vi "SCMP FITS - Make Single FITS Header.vi"(6 "FITS info":T4={"File name"="lsob_demo_0530_LM_20190529_124525_live_C1_00020_001_lev0.0.fits", "Date"="2019-05-29T12:45:25"}, 7 "Andor":T1={"Handle"=0, "Pixel Encoding"="", "AOI Width"=0, "AOI Height"=0, "AOI Stride"=0, "Row Readout Time"=0.0, "Frame Readout Time"=0.0, "Interframe Time"=0.0, "Semaphore"=refnum, "SerialNumber"="", "Camera Model"="", "Controller ID"="", "Firmware Version"="", "Shutter"="Global", "BDiv"=1, "Time at Synch"=timestamp(3029526000.379448 s since 1904-01-01), "Idx"=0, "PreAmp"="", "Binning"=enum."1x1", "PixelReadoutRate"="", "Exposure (s)"=0.05, "Image Bytes"=0, "Image Pixels"=0, "SpuriousNoiseFilter"=FALSE, "Overlap"=FALSE, "CycleMode"=""} {"Exposure (s)" format="%^.3g"; "Time at Synch" format="%<%H:%M:%S>T"; "Interframe Time" format="%#_3g"; "Frame Readout Time" format="%_3g"; "Row Readout Time" format="%_3g"}, 8 "error in":errorcluster, 9 "NAXIS":string="2", 10 "FITS Header":T5={"Wavelength (nm)"=530.15, "Exposure (s)"=0.05, "Tuning Delay (ms)"=1000.0, "Beam Type (-1/1)"=1.0, "Tuning Voltages"=[1.111, 2.222, 3.333, 4.444], "Observer"="observer", "Light Shapping Diffuser"=enum."In Beam", "Comment"="", "Data Type"=enum."HOLE", "Mod Cycles"=0, "SCD Calibration Optics"=enum."1 - Polarizer @0, I+Q", "SCD Emission Line Filter"=enum."1-557.6nm", "Cookbook"="", "COMP-S Calibration Wheel"=enum."Dark", "COMP-S Andover Filter Wheel"=enum."530.3nm/HWB 0.34nm (Fe XIV)", "FOV Rotation (deg)"=66.0, "Objective Lens Position (mm)"=0.0, "Occulter size"=0.0, "Time End"=timestamp(3382374145.421875 s since 1904-01-01), "Acc Exposure (s)"=0.0, "Time Stamp Array"=[], "Camera Serial Number"=[], "Camera Temp"=[], "Camera PI (mm)"=[], "Time Start"=timestamp(3382374145.421875 s since 1904-01-01), "Peripherals"={"ILX controler"=FALSE, "Zone temperatures"=FALSE, "Andor"=FALSE, "Andor 2"=FALSE, "PI Stages"=FALSE, "AISAS mechanisms"=FALSE, "AISAS Mech.lvclass"=refnum, "Zone temp ref"=variant, "FWs"=FALSE}, "FITS paths"=[], "Cameras"=enum."Andor", "load preset cbk"=FALSE, "periodic check count"=0, "COMP-S Calibration Wheel 2"=enum."Dark", "Calib"=enum."Dark", "Abso Aperture"=66.0, "Nominal Aperture"=66.0} {"Nominal Aperture" format="%.1f"; "Abso Aperture" format="%.1f"; "Camera PI (mm)" format="%_3g"; "Acc Exposure (s)" format="%^.3g"; "Occulter size" format="%.2f"; "Objective Lens Position (mm)" min=70.0 max=152.0 format="%.2f"; "FOV Rotation (deg)" format="%.1f"; "Exposure (s)" format="%^.3g"; "Wavelength (nm)" format="%_6g"}, 11 "Image #":i32) -> (0 "error out":errorcluster, 1 "23040 Byte Header":string="SIMPLE  =                              T / CONFORMS TO FITS STANDARD            BITPIX  =                             32 / BITS PER PIXEL                       NAXIS   =                              2 / DATA DIMENSIONS IN FITS FILE         NAXIS1  =                              0 / XDIM (PIXELS)                        NAXIS2  =                              0 / YDIM (PIXELS)                        NAXIS3  =                              4 / 4 POLARIZATION STATES                NAXIS4  =                              1 / 1 CAMERA                             ORIGIN  =                        'AISAS' / SCIENTIFIC GROUP                     OBSERVER=                     'SCHWARTZ' / NAME OF OBSERVER                     TELESCOP=                   '20CM ZEISS' / NAME OF TELESCOPE                    LOCATION=            'LOMNICKY PEAK OBS' / LOCATION OF TELESCOPE                INSTRUME=                          'SCD' / NAME OF INSTRUMENT                   BZERO   =                             0. /  ADU OFFSET                          FOCUS   =                             26 / CAMERA-STAGE POSITION (MM)           ROTPOS  =                           66.0 / ROTATIONAL POSITION (DEG)            DIFFUSER=                      'IN BEAM' / 0=IN BEAM, 1=OUT OF BEAM             FW-WVLNG=                        '557.6' / PRE-FILTER CENTER WAVELENGTH (NM)    FW-CALIB=                         'DARK' / CAL-WHEEL POSITION                   CAM-SN1 =                    'SCC-02209' / CAMERA SERIAL NUMBER                 CAM-TEMP=                       0.000000 / FOCAL PLANE TEMP (C)                 TUNEDLAY=                           1000 / LCVR RELAXATION DELAY (mS)           DATE_OBS=                     '3/7/2011' / DATE OF OBSERVATION START (UTC)      TIME_OBS=                   '212225.421' / TIME OF OBSERVATION (UTC)            EXPOSURE=                       0.050000 / EXPOSURE TIME (S)                    MODC    =                              0 / NUMBER OF IMAGES AT EACH STATE       NLC-1   =                          1.111 / TUNING VOLTAGE-1                     NLC-2   =                          2.222 / TUNING VOLTAGE-2                     NLC-3   =                          3.333 / TUNING VOLTAGE-3                     NLC-4   =                          4.444 / TUNING VOLTAGE-4                     NLC-5   =                          0.000 / TUNING VOLTAGE-5                     BEAM    =                              1 / BEAM (0=ON BAND OR 1=CONTINUUM)      WAVELENG=                         530.15 / WAVELENGTH OF OBS (NM)               COMMHEAD=                             '' / OBSERVER COMMENT                     COOKBOOK=                                / COOKBOOK  LOADED                     COMMENT                                                                         COMMENT                                                                         COMMENT                                                                         COMMENT                                                                         COMMENT                                                                         COMMENT                                                                         COMMENT                                                                         COMMENT                                                                         COMMENT                                                                         COMMENT                                                                         COMMENT                                                                         COMMENT                                                                         COMMENT                                                                         COMMENT                                                                         COMMENT                                                                         COMMENT                                                                         COMMENT                                                                         COMMENT                                                                         COMMENT                                                                         COMMENT                                                                         COMMENT                                                                         COMMENT                                                                         COMMENT                                                                         COMMENT                                                                         COMMENT                                                                         COMMENT                                                                         COMMENT                                                                         COMMENT                                                                         COMMENT                                                                         COMMENT                                                                         COMMENT                                                                         COMMENT                                                                         COMMENT                                                                         COMMENT                                                                         COMMENT                                                                         COMMENT                                                                         COMMENT                                                                         COMMENT                                                                         COMMENT                                                                         COMMENT                                                                         COMMENT                                                                         COMMENT                                                                         COMMENT                                                                         COMMENT                                                                         COMMENT                                                                         COMMENT                                                                         COMMENT                                                                         COMMENT                                                                         COMMENT                                                                         COMMENT                                                                         COMMENT                                                                         COMMENT                                                                         COMMENT                                                                         COMMENT                                                                         COMMENT                                                                         COMMENT                                                                         COMMENT                                                                         COMMENT                                                                         COMMENT                                                                         COMMENT                                                                         COMMENT                                                                         COMMENT                                                                         COMMENT                                                                         COMMENT                                                                         COMMENT                                                                         COMMENT                                                                         COMMENT                                                                         COMMENT                                                                         COMMENT                                                                         COMMENT                                                                         COMMENT                                                                         COMMENT                                                                         COMMENT                                                                         COMMENT                                                                         COMMENT                                                                         COMMENT                                                                         COMMENT                                                                         COMMENT                                                                         COMMENT                                                                         COMMENT                                                                         COMMENT                                                                         COMMENT                                                                         COMMENT                                                                         COMMENT                                                                         COMMENT                                                                         COMMENT                                                                         COMMENT                                                                         COMMENT                                                                         COMMENT                                                                         COMMENT                                                                         COMMENT                                                                         COMMENT                                                                         COMMENT                                                                         COMMENT                                                                         COMMENT                                                                         COMMENT                                                                         COMMENT                                                                         COMMENT                                                                         COMMENT                                                                         COMMENT                                                                         COMMENT                                                                         COMMENT                                                                         COMMENT                                                                         COMMENT                                                                         COMMENT                                                                         COMMENT                                                                         COMMENT                                                                         COMMENT                                                                         COMMENT                                                                         COMMENT                                                                         COMMENT                                                                         COMMENT                                                                         COMMENT                                                                         COMMENT                                                                         COMMENT                                                                         COMMENT                                                                         COMMENT                                                                         COMMENT                                                                         COMMENT                                                                         COMMENT                                                                         COMMENT                                                                         COMMENT                                                                         COMMENT                                                                         COMMENT                                                                         COMMENT                                                                         COMMENT                                                                         COMMENT                                                                         COMMENT                                                                         COMMENT                                                                         COMMENT                                                                         COMMENT                                                                         COMMENT                                                                         COMMENT                                                                         COMMENT                                                                         COMMENT                                                                         COMMENT                                                                         COMMENT                                                                         COMMENT                                                                         COMMENT                                                                         COMMENT                                                                         COMMENT                                                                         COMMENT                                                                         COMMENT                                                                         COMMENT                                                                         COMMENT                                                                         COMMENT                                                                         COMMENT                                                                         COMMENT                                                                         COMMENT                                                                         COMMENT                                                                         COMMENT                                                                         COMMENT                                                                         COMMENT                                                                         COMMENT                                                                         COMMENT                                                                         COMMENT                                                                         COMMENT                                                                         COMMENT                                                                         COMMENT                                                                         COMMENT                                                                         COMMENT                                                                         COMMENT                                                                         COMMENT                                                                         COMMENT                                                                         COMMENT                                                                         COMMENT                                                                         COMMENT                                                                         COMMENT                                                                         COMMENT                                                                         COMMENT                                                                         COMMENT                                                                         COMMENT                                                                         COMMENT                                                                         COMMENT                                                                         COMMENT                                                                         COMMENT                                                                         COMMENT                                                                         COMMENT                                                                         COMMENT                                                                         COMMENT                                                                         COMMENT                                                                         COMMENT                                                                         COMMENT                                                                         COMMENT                                                                         COMMENT                                                                         COMMENT                                                                         COMMENT                                                                         COMMENT                                                                         COMMENT                                                                         COMMENT                                                                         COMMENT                                                                         COMMENT                                                                         COMMENT                                                                         COMMENT                                                                         COMMENT                                                                         COMMENT                                                                         COMMENT                                                                         COMMENT                                                                         COMMENT                                                                         COMMENT                                                                         COMMENT                                                                         COMMENT                                                                         COMMENT                                                                         COMMENT                                                                         COMMENT                                                                         COMMENT                                                                         COMMENT                                                                         COMMENT                                                                         COMMENT                                                                         COMMENT                                                                         COMMENT                                                                         COMMENT                                                                         COMMENT                                                                         COMMENT                                                                         COMMENT                                                                         COMMENT                                                                         COMMENT                                                                         COMMENT                                                                         COMMENT                                                                         COMMENT                                                                         COMMENT                                                                         COMMENT                                                                         COMMENT                                                                         COMMENT                                                                         COMMENT                                                                         COMMENT                                                                         COMMENT                                                                         COMMENT                                                                         COMMENT                                                                         COMMENT                                                                         COMMENT                                                                         COMMENT                                                                         COMMENT                                                                         COMMENT                                                                         COMMENT                                                                         COMMENT                                                                         COMMENT                                                                         COMMENT                                                                         COMMENT                                                                         COMMENT                                                                         COMMENT                                                                         COMMENT                                                                         COMMENT                                                                         COMMENT                                                                         COMMENT                                                                         COMMENT                                                                         COMMENT                                                                         COMMENT                                                                         COMMENT                                                                         COMMENT                                                                         COMMENT                                                                         COMMENT                                                                         COMMENT                                                                         END                                                                             ", 3 "final header byte length":i32=23040)   [LabVIEW 2014]
uses:
  Controls/SCD - FITS Cluster.ctl
  AISAS/Mech/AISAS Mech.lvclass
  AISAS/Controls/Diffuser.ctl
  Controls/FITS Data type.ctl
  Controls/SCD - Calibration Optics Filter Wheel.ctl
  Controls/SCD - EDT - Emission Line Filter Wheel.ctl
  Controls/CoMP-S Controls/Polarization Optics Filter Wheel.ctl
  Controls/CoMP-S Controls/Emission Line Filter Wheel.ctl
  AISAS/Controls/focus.ctl
  Controls/peripherals.ctl
  Controls/Cameras select.ctl
  Controls/Fits info.ctl
  Camera/Andor Neo Info.ctl
  Controls/beaning.ctl
  Controls/Globals.vi
panel:
  out "Required COMMENT Rows":i32
  in  "NAXIS2":string="2160"
  in  "NAXIS1":string="2560"
  out "Header Rows":i32=34
  out "FITS Header":string[](array[string])=["SIMPLE  =                              T / CONFORMS TO FITS STANDARD            ", "BITPIX  =                             32 / BITS PER PIXEL                       ", "NAXIS   =                              2 / DATA DIMENSIONS IN FITS FILE         ", "NAXIS1  =                              0 / XDIM (PIXELS)                        ", "NAXIS2  =                              0 / YDIM (PIXELS)                        ", "NAXIS3  =                              4 / 4 POLARIZATION STATES                ", "NAXIS4  =                              1 / 1 CAMERA                             ", "ORIGIN  =                        'AISAS' / SCIENTIFIC GROUP                     ", "OBSERVER=                     'SCHWARTZ' / NAME OF OBSERVER                     ", "TELESCOP=                   '20CM ZEISS' / NAME OF TELESCOPE                    ", "LOCATION=            'LOMNICKY PEAK OBS' / LOCATION OF TELESCOPE                ", "INSTRUME=                          'SCD' / NAME OF INSTRUMENT                   ", "BZERO   =                             0. /  ADU OFFSET                          ", "FOCUS   =                             26 / CAMERA-STAGE POSITION (MM)           ", "ROTPOS  =                           66.0 / ROTATIONAL POSITION (DEG)            ", "DIFFUSER=                      'IN BEAM' / 0=IN BEAM, 1=OUT OF BEAM             ", "FW-WVLNG=                        '557.6' / PRE-FILTER CENTER WAVELENGTH (NM)    ", "FW-CALIB=                         'DARK' / CAL-WHEEL POSITION                   ", "CAM-SN1 =                    'SCC-02209' / CAMERA SERIAL NUMBER                 ", "CAM-TEMP=                       0.000000 / FOCAL PLANE TEMP (C)                 ", "TUNEDLAY=                           1000 / LCVR RELAXATION DELAY (mS)           ", "DATE_OBS=                     '3/7/2011' / DATE OF OBSERVATION START (UTC)      ", "TIME_OBS=                   '212225.421' / TIME OF OBSERVATION (UTC)            ", "EXPOSURE=                       0.050000 / EXPOSURE TIME (S)                    ", "MODC    =                              0 / NUMBER OF IMAGES AT EACH STATE       ", "NLC-1   =                          1.111 / TUNING VOLTAGE-1                     ", "NLC-2   =                          2.222 / TUNING VOLTAGE-2                     ", "NLC-3   =                          3.333 / TUNING VOLTAGE-3                     ", "NLC-4   =                          4.444 / TUNING VOLTAGE-4                     ", "NLC-5   =                          0.000 / TUNING VOLTAGE-5                     ", "BEAM    =                              1 / BEAM (0=ON BAND OR 1=CONTINUUM)      ", "WAVELENG=                         530.15 / WAVELENGTH OF OBS (NM)               ", "COMMHEAD=                             '' / OBSERVER COMMENT                     ", "COOKBOOK=                                / COOKBOOK  LOADED                     ", "COMMENT                                                                         ", "COMMENT                                                                         ", "COMMENT                                                                         ", "COMMENT                                                                         ", "COMMENT                                                                         ", "COMMENT                                                                         ", "COMMENT                                                                         ", "COMMENT                                                                         ", "COMMENT                                                                         ", "COMMENT                                                                         ", "COMMENT                                                                         ", "COMMENT                                                                         ", "COMMENT                                                                         ", "COMMENT                                                                         ", "COMMENT                                                                         ", "COMMENT                                                                         ", "COMMENT                                                                         ", "COMMENT                                                                         ", "COMMENT                                                                         ", "COMMENT                                                                         ", "COMMENT                                                                         ", "COMMENT                                                                         ", "COMMENT                                                                         ", "COMMENT                                                                         ", "COMMENT                                                                         ", "COMMENT                                                                         ", "COMMENT                                                                         ", "COMMENT                                                                         ", "COMMENT                                                                         ", "COMMENT                                                                         ", "COMMENT                                                                         ", "COMMENT                                                                         ", "COMMENT                                                                         ", "COMMENT                                                                         ", "COMMENT                                                                         ", "COMMENT                                                                         ", "COMMENT                                                                         ", "COMMENT                                                                         ", "COMMENT                                                                         ", "COMMENT                                                                         ", "COMMENT                                                                         ", "COMMENT                                                                         ", "COMMENT                                                                         ", "COMMENT                                                                         ", "COMMENT                                                                         ", "COMMENT                                                                         ", "COMMENT                                                                         ", "COMMENT                                                                         ", "COMMENT                                                                         ", "COMMENT                                                                         ", "COMMENT                                                                         ", "COMMENT                                                                         ", "COMMENT                                                                         ", "COMMENT                                                                         ", "COMMENT                                                                         ", "COMMENT                                                                         ", "COMMENT                                                                         ", "COMMENT                                                                         ", "COMMENT                                                                         ", "COMMENT                                                                         ", "COMMENT                                                                         ", "COMMENT                                                                         ", "COMMENT                                                                         ", "COMMENT                                                                         ", "COMMENT                                                                         ", "COMMENT                                                                         ", "COMMENT                                                                         ", "COMMENT                                                                         ", "COMMENT                                                                         ", "COMMENT                                                                         ", "COMMENT                                                                         ", "COMMENT                                                                         ", "COMMENT                                                                         ", "COMMENT                                                                         ", "COMMENT                                                                         ", "COMMENT                                                                         ", "COMMENT                                                                         ", "COMMENT                                                                         ", "COMMENT                                                                         ", "COMMENT                                                                         ", "COMMENT                                                                         ", "COMMENT                                                                         ", "COMMENT                                                                         ", "COMMENT                                                                         ", "COMMENT                                                                         ", "COMMENT                                                                         ", "COMMENT                                                                         ", "COMMENT                                                                         ", "COMMENT                                                                         ", "COMMENT                                                                         ", "COMMENT                                                                         ", "COMMENT                                                                         ", "COMMENT                                                                         ", "COMMENT                                                                         ", "COMMENT                                                                         ", "COMMENT                                                                         ", "COMMENT                                                                         ", "COMMENT                                                                         ", "COMMENT                                                                         ", "COMMENT                                                                         ", "COMMENT                                                                         ", "COMMENT                                                                         ", "COMMENT                                                                         ", "COMMENT                                                                         ", "COMMENT                                                                         ", "COMMENT                                                                         ", "COMMENT                                                                         ", "COMMENT                                                                         ", "COMMENT                                                                         ", "COMMENT                                                                         ", "COMMENT                                                                         ", "COMMENT                                                                         ", "COMMENT                                                                         ", "COMMENT                                                                         ", "COMMENT                                                                         ", "COMMENT                                                                         ", "COMMENT                                                                         ", "COMMENT                                                                         ", "COMMENT                                                                         ", "COMMENT                                                                         ", "COMMENT                                                                         ", "COMMENT                                                                         ", "COMMENT                                                                         ", "COMMENT                                                                         ", "COMMENT                                                                         ", "COMMENT                                                                         ", "COMMENT                                                                         ", "COMMENT                                                                         ", "COMMENT                                                                         ", "COMMENT                                                                         ", "COMMENT                                                                         ", "COMMENT                                                                         ", "COMMENT                                                                         ", "COMMENT                                                                         ", "COMMENT                                                                         ", "COMMENT                                                                         ", "COMMENT                                                                         ", "COMMENT                                                                         ", "COMMENT                                                                         ", "COMMENT                                                                         ", "COMMENT                                                                         ", "COMMENT                                                                         ", "COMMENT                                                                         ", "COMMENT                                                                         ", "COMMENT                                                                         ", "COMMENT                                                                         ", "COMMENT                                                                         ", "COMMENT                                                                         ", "COMMENT                                                                         ", "COMMENT                                                                         ", "COMMENT                                                                         ", "COMMENT                                                                         ", "COMMENT                                                                         ", "COMMENT                                                                         ", "COMMENT                                                                         ", "COMMENT                                                                         ", "COMMENT                                                                         ", "COMMENT                                                                         ", "COMMENT                                                                         ", "COMMENT                                                                         ", "COMMENT                                                                         ", "COMMENT                                                                         ", "COMMENT                                                                         ", "COMMENT                                                                         ", "COMMENT                                                                         ", "COMMENT                                                                         ", "COMMENT                                                                         ", "COMMENT                                                                         ", "COMMENT                                                                         ", "COMMENT                                                                         ", "COMMENT                                                                         ", "COMMENT                                                                         ", "COMMENT                                                                         ", "COMMENT                                                                         ", "COMMENT                                                                         ", "COMMENT                                                                         ", "COMMENT                                                                         ", "COMMENT                                                                         ", "COMMENT                                                                         ", "COMMENT                                                                         ", "COMMENT                                                                         ", "COMMENT                                                                         ", "COMMENT                                                                         ", "COMMENT                                                                         ", "COMMENT                                                                         ", "COMMENT                                                                         ", "COMMENT                                                                         ", "COMMENT                                                                         ", "COMMENT                                                                         ", "COMMENT                                                                         ", "COMMENT                                                                         ", "COMMENT                                                                         ", "COMMENT                                                                         ", "COMMENT                                                                         ", "COMMENT                                                                         ", "COMMENT                                                                         ", "COMMENT                                                                         ", "COMMENT                                                                         ", "COMMENT                                                                         ", "COMMENT                                                                         ", "COMMENT                                                                         ", "COMMENT                                                                         ", "COMMENT                                                                         ", "COMMENT                                                                         ", "COMMENT                                                                         ", "COMMENT                                                                         ", "COMMENT                                                                         ", "COMMENT                                                                         ", "COMMENT                                                                         ", "COMMENT                                                                         ", "COMMENT                                                                         ", "COMMENT                                                                         ", "COMMENT                                                                         ", "COMMENT                                                                         ", "COMMENT                                                                         ", "COMMENT                                                                         ", "COMMENT                                                                         ", "COMMENT                                                                         ", "COMMENT                                                                         ", "COMMENT                                                                         ", "COMMENT                                                                         ", "COMMENT                                                                         ", "COMMENT                                                                         ", "COMMENT                                                                         ", "COMMENT                                                                         ", "COMMENT                                                                         ", "COMMENT                                                                         ", "COMMENT                                                                         ", "COMMENT                                                                         ", "COMMENT                                                                         ", "COMMENT                                                                         ", "COMMENT                                                                         ", "COMMENT                                                                         ", "COMMENT                                                                         ", "COMMENT                                                                         ", "COMMENT                                                                         ", "COMMENT                                                                         ", "COMMENT                                                                         ", "COMMENT                                                                         ", "COMMENT                                                                         ", "COMMENT                                                                         ", "COMMENT                                                                         ", "COMMENT                                                                         ", "COMMENT                                                                         ", "COMMENT                                                                         ", "COMMENT                                                                         ", "COMMENT                                                                         ", "COMMENT                                                                         ", "COMMENT                                                                         ", "COMMENT                                                                         ", "COMMENT                                                                         ", "COMMENT                                                                         ", "COMMENT                                                                         ", "END                                                                             "]
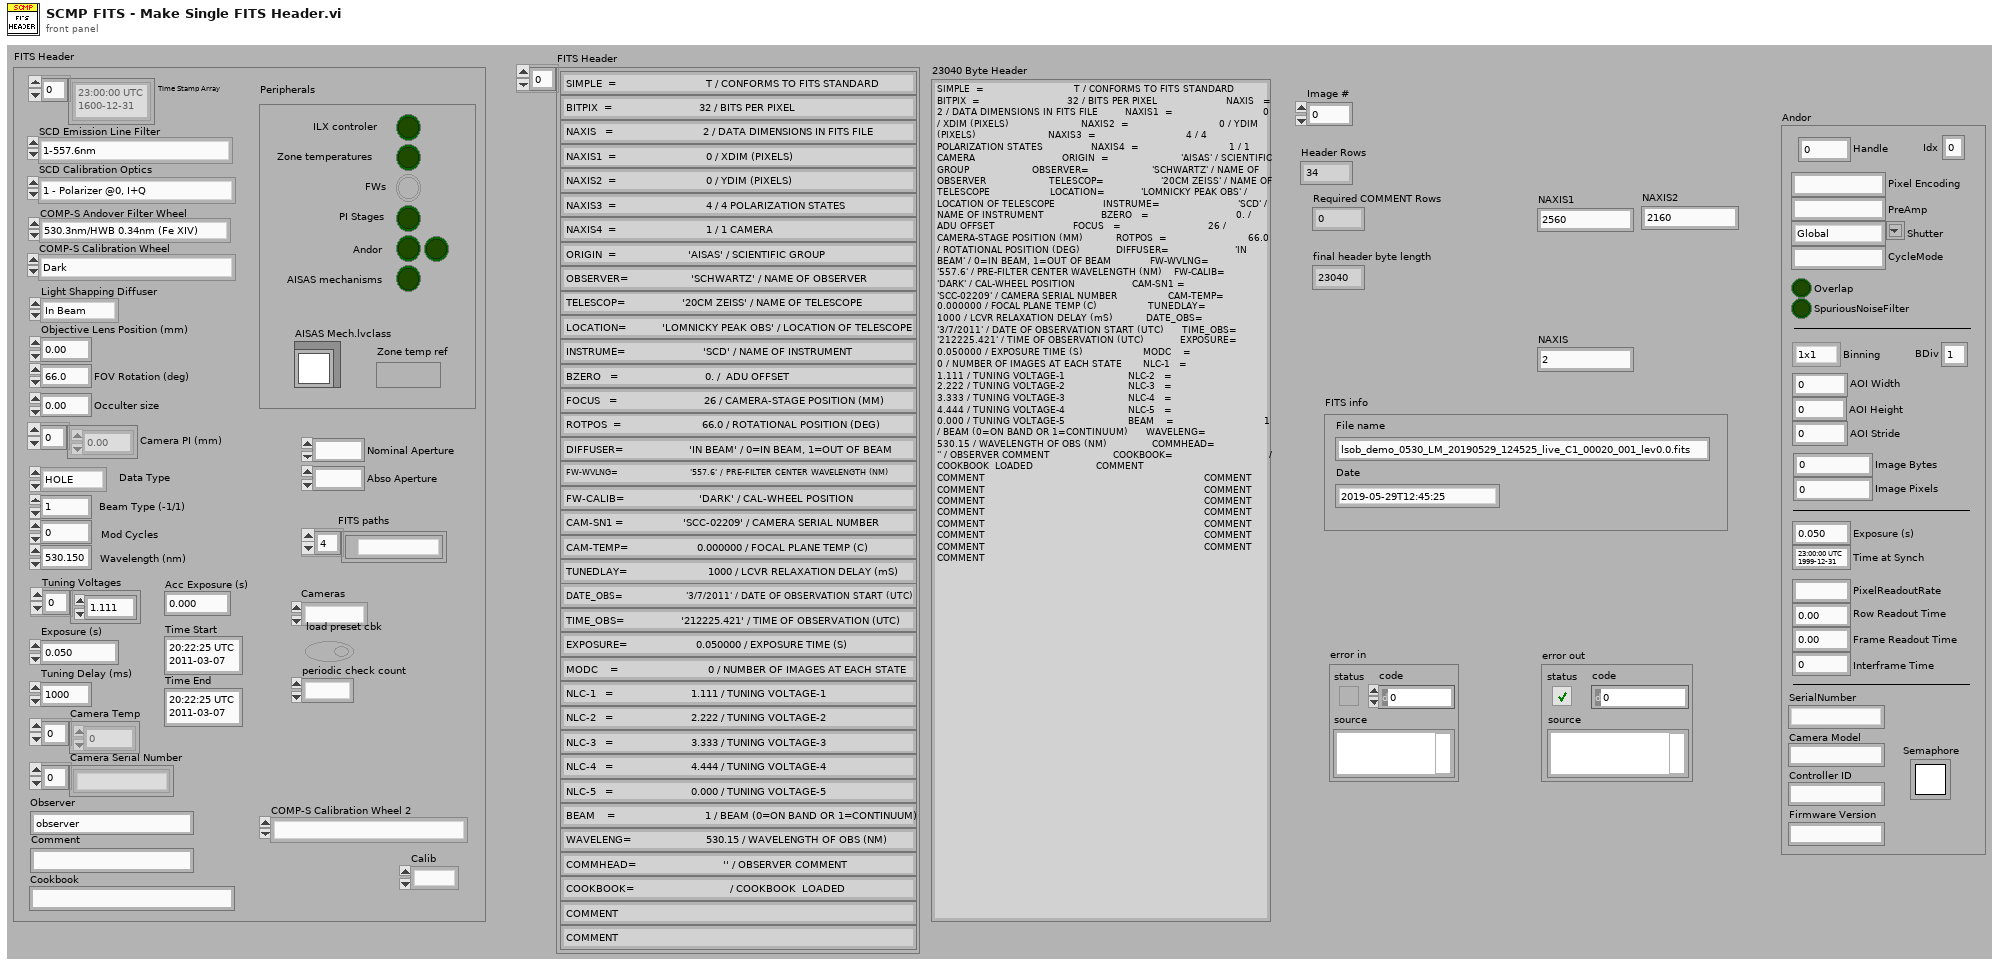
[diagram p1: front panel]
types:
  T1 = typedef "Andor Neo Info.ctl" = cluster{"Handle":i32, "Pixel Encoding":string, "AOI Width":i32, "AOI Height":i32, "AOI Stride":i32, "Row Readout Time":dbl, "Frame Readout Time":dbl, "Interframe Time":dbl, "Semaphore":T2, "SerialNumber":string, "Camera Model":string, "Controller ID":string, "Firmware Version":string, "Shutter":string, "BDiv":u8, "Time at Synch":timestamp, "Idx":i32, "PreAmp":string, "Binning":T3, "PixelReadoutRate":string, "Exposure (s)":dbl, "Image Bytes":i64, "Image Pixels":i64, "SpuriousNoiseFilter":bool, "Overlap":bool, "CycleMode":string}
  T2 = typedef "Semaphore RefNum" = refnum<k1>
  T3 = typedef "beaning.ctl" = enum16{"1x1", "2x2", "3x3", "4x4", "8x8"}
  T4 = typedef "Fits info.ctl" = cluster{"File name":string, "Date":string}
  T5 = typedef "SCD - FITS Cluster.ctl" = cluster{"Wavelength (nm)":dbl, "Exposure (s)":dbl, "Tuning Delay (ms)":dbl, "Beam Type (-1/1)":dbl, "Tuning Voltages":dbl[], "Observer":string, "Light Shapping Diffuser":T6, "Comment":string, "Data Type":T7, "Mod Cycles":u16, "SCD Calibration Optics":T8, "SCD Emission Line Filter":T9, "Cookbook":string, "COMP-S Calibration Wheel":T10, "COMP-S Andover Filter Wheel":T11, "FOV Rotation (deg)":dbl, "Objective Lens Position (mm)":T12, "Occulter size":dbl, "Time End":timestamp, "Acc Exposure (s)":dbl, "Time Stamp Array":timestamp[], "Camera Serial Number":string[], "Camera Temp":dbl[], "Camera PI (mm)":dbl[], "Time Start":timestamp, "Peripherals":T13, "FITS paths":path[], "Cameras":T14, "load preset cbk":bool, "periodic check count":i32, "COMP-S Calibration Wheel 2":T10, "Calib":enum16{"Dark", "Flat"}, "Abso Aperture":dbl, "Nominal Aperture":dbl}
  T6 = typedef "Diffuser.ctl" = enum16{"Out of Beam", "In Beam"}
  T7 = typedef "FITS Data type.ctl" = enum16{"LIVE", "DARK", "FLAT", "CALI", "OBSE", "ABSO", "AURE", "TARG", "OBJE", "HOLE", "OREX", "THRO", "CHIP"}
  T8 = typedef "SCD - Calibration Optics Filter Wheel.ctl" = enum16{"1 - Polarizer @0, I+Q", "2 - Polarizer @90, I-Q", "3 - Polarizer @45, I+U", "4 - Polarizer @135, I-U", "5 - Polarizer @0, Retarder @45, I+V", "6 - Polarizer @0, Retarder @135, I-V", "7 - Dark", "8 - Clear", "9 - N/A"}
  T9 = typedef "SCD - EDT - Emission Line Filter Wheel.ctl" = enum16{"1-557.6nm", "2-587.6nm", "3-589.6nm", "4-630.2nm", "5-656.4nm", "6-849.8nm", "7-854.2nm", "8-866.2nm", "9-1083.0nm"}
  T10 = typedef "Polarization Optics Filter Wheel.ctl" = enum16{"Dark", "Clear", "Exchange Lens", "Polarizer @0, I+Q", "Polarizer @90, I-Q", "Polarizer @45, I+U", "Polarizer @135, I-U", "Polarizer @0, Retarder @45, I+V", "Polarizer @0, Retarder @135, I-V"}
  T11 = typedef "Emission Line Filter Wheel.ctl" = enum16{"530.3nm/HWB 0.34nm (Fe XIV)", "587.6nm/HBW 0.44nm (He I D3)", "637.5nm/HBW 0.53nm (Fe X)", "656.3nm/HBW 0.57nm (H-Alpha)", "789.2nm/HBW 0.85nm (Fe XI)", "854.2nm/HBW 1.01nm (Ca I)", "1074.7nm/HBW 2.34nm (Fe XIII)", "1079.8nm/HBW 1.64nm (Fe XIII)", "1083.0nm/HBW 1.66nm (He I)"}
  T12 = typedef "focus.ctl" = dbl
  T13 = typedef "peripherals.ctl" = cluster{"ILX controler":bool, "Zone temperatures":bool, "Andor":bool, "Andor 2":bool, "PI Stages":bool, "AISAS mechanisms":bool, "AISAS Mech.lvclass":refnum<class "AISAS Mech.lvclass">, "Zone temp ref":variant, "FWs":bool}
  T14 = typedef "Cameras select.ctl" = enum16{"Andor", "GDR"}
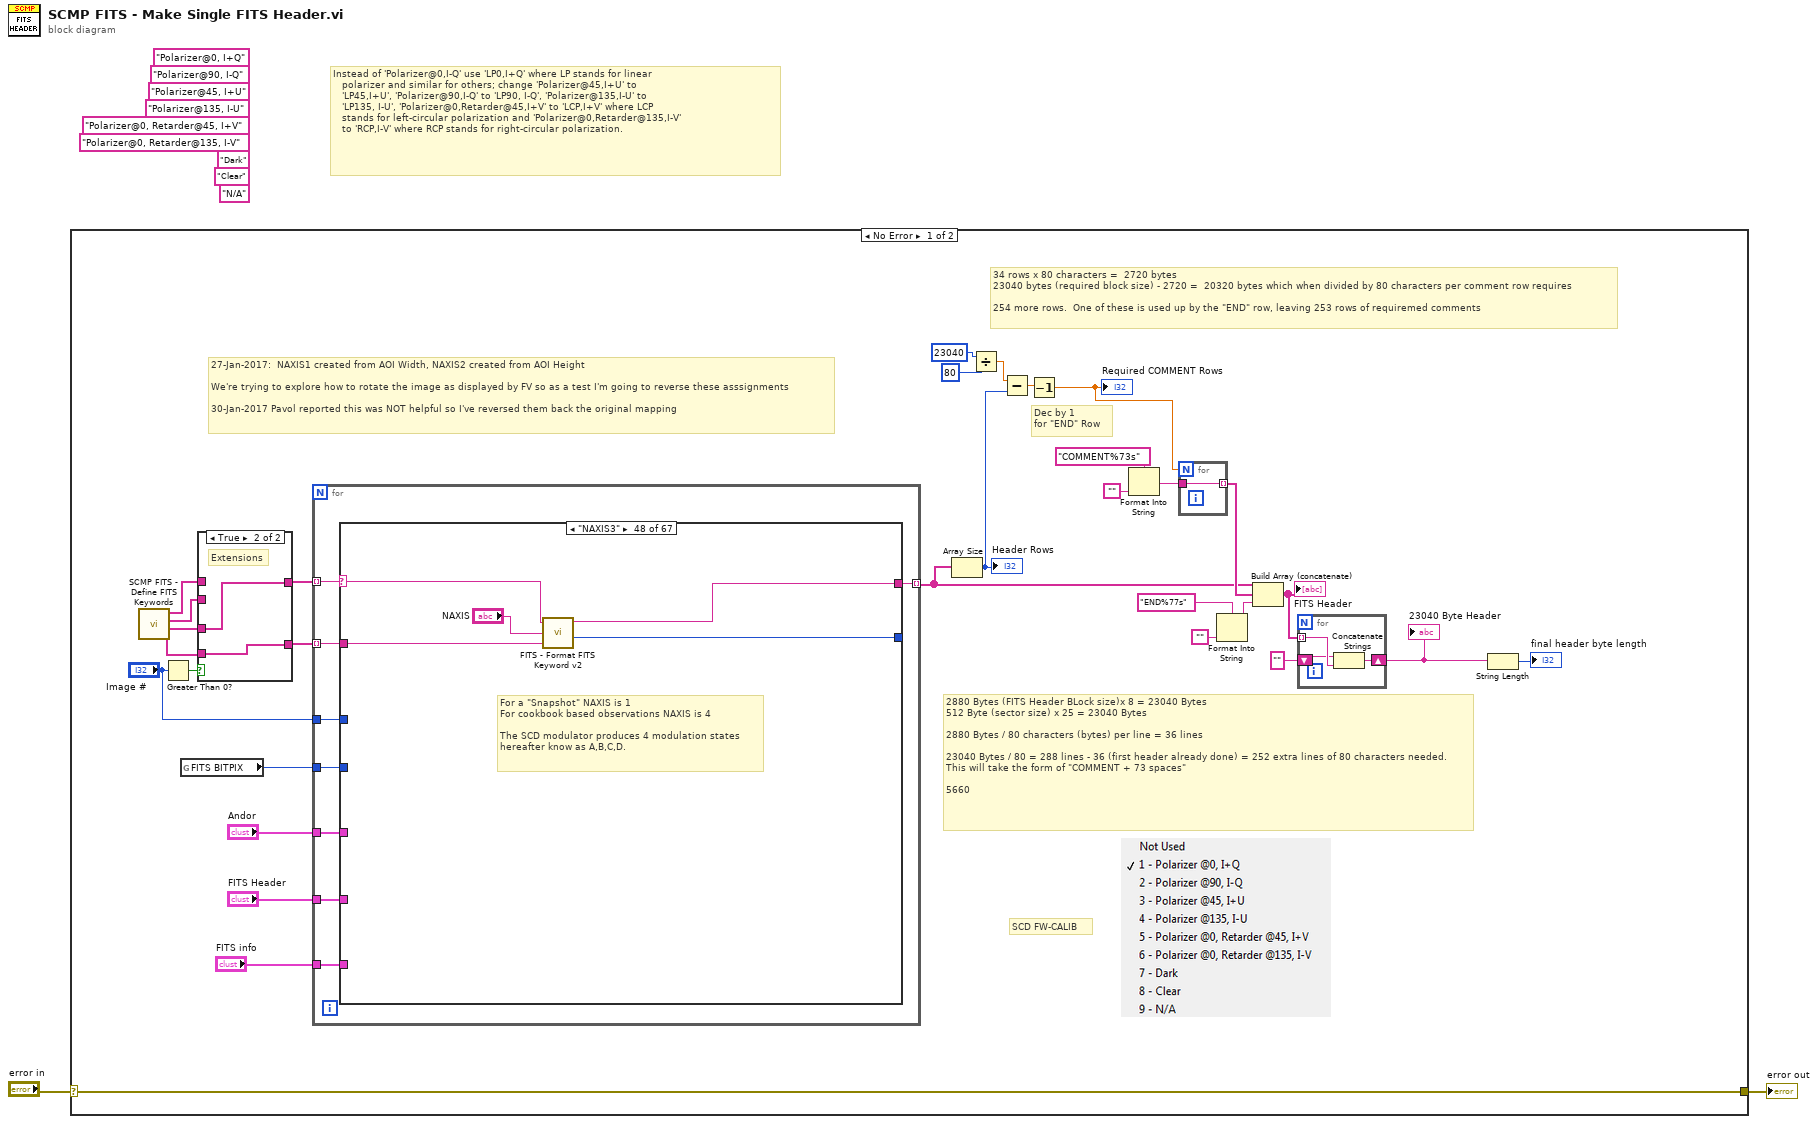
[diagram p0: block diagram]
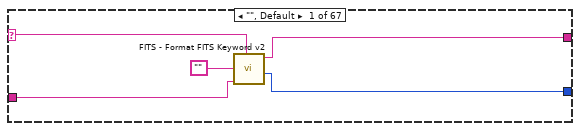
[diagram p3: hidden frame]
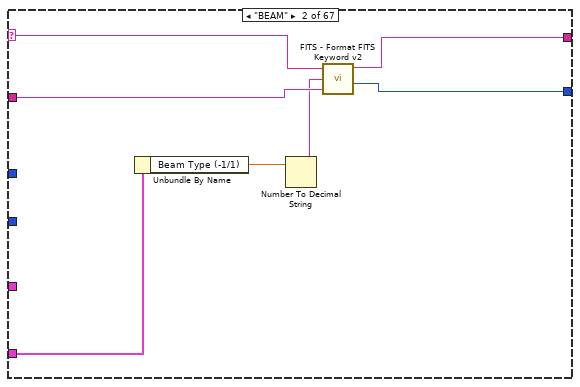
[diagram p4: hidden frame]
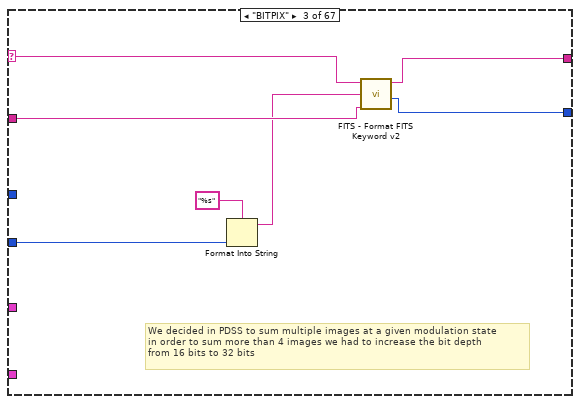
[diagram p5: hidden frame]
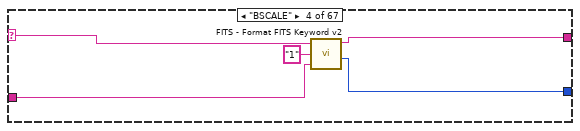
[diagram p6: hidden frame]
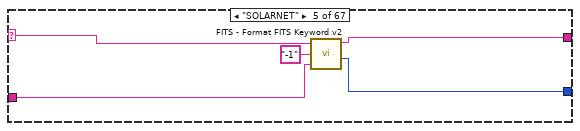
[diagram p7: hidden frame]
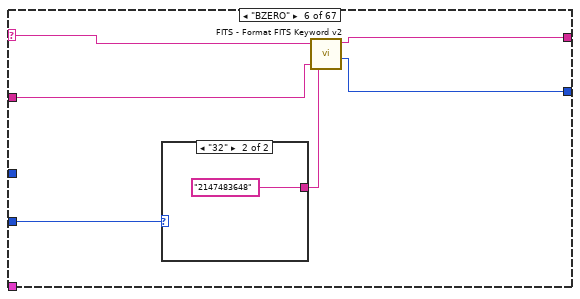
[diagram p8: hidden frame]
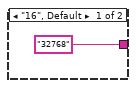
[diagram p9: hidden frame]
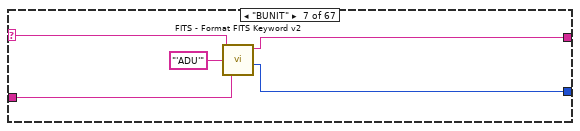
[diagram p10: hidden frame]
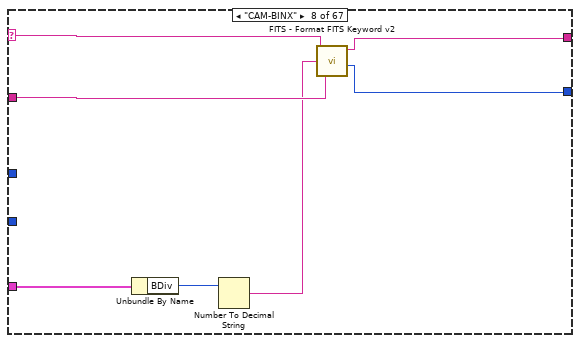
[diagram p11: hidden frame]
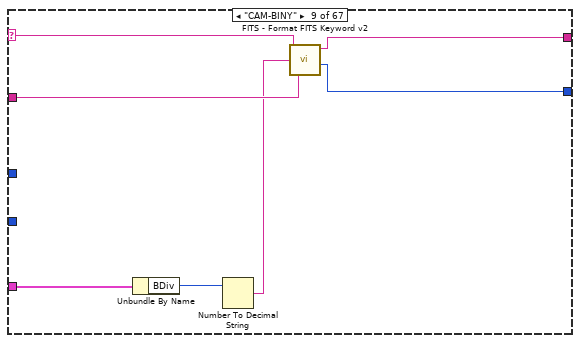
[diagram p12: hidden frame]
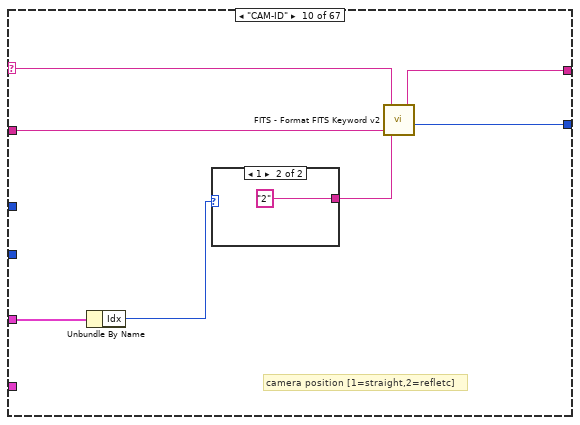
[diagram p13: hidden frame]
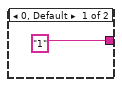
[diagram p14: hidden frame]
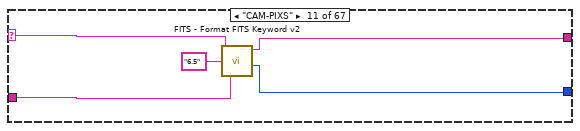
[diagram p15: hidden frame]
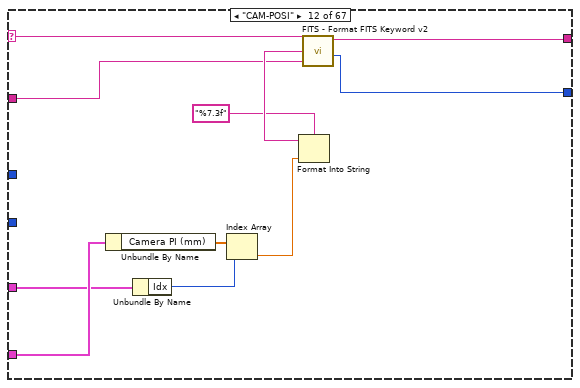
[diagram p16: hidden frame]
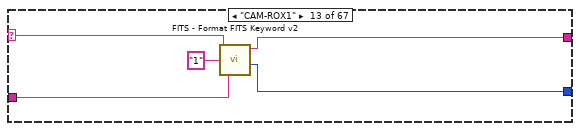
[diagram p17: hidden frame]
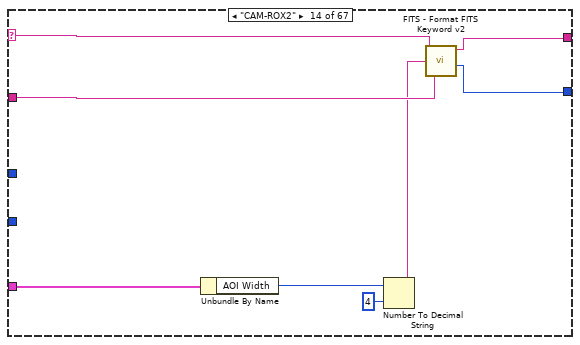
[diagram p18: hidden frame]
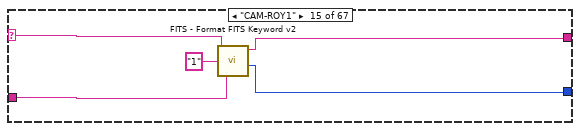
[diagram p19: hidden frame]
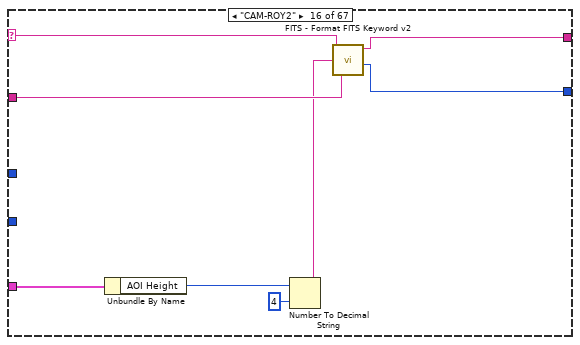
[diagram p20: hidden frame]
diagram:
  (unwired) "N/A" ("element")
  (unwired) "Clear" ("element")
  (unwired) "Dark" ("element")
  (unwired) "Polarizer@0, Retarder@135, I-V" ("element")
  (unwired) "Polarizer@0, Retarder@45, I+V" ("element")
  (unwired) "Polarizer@135, I-U" ("element")
  (unwired) "Polarizer@45, I+U"
  (unwired) "Polarizer@90, I-Q"
  (unwired) "Polarizer@0, I+Q"
  # "Instead of 'Polarizer@0,I-Q' use 'LP0,I+Q' where LP stands for linear\n   polarizer and similar for others; change 'Polarizer@45,I+U' to\n   'LP45,I+U', 'Polarizer@90,I-Q' to 'LP90, I-Q', 'Polarizer@135,I-U' to\n   'LP135, I-U', 'Polarizer@0,Retarder@45,I+V' to 'LCP,I+V' where LCP\n   stands for left-circular polarization and 'Polarizer@0,Retarder@135,I-V'\n   to 'RCP,I-V' where RCP stands for right-circular polarization."
  n1 = case shown="No Error" "error in" {
    selector: "error in" -> [w14 w605]
    tunnel: [w14 w605] -> w1
    frame No Error {
      # "SCD FW-CALIB"
      # "27-Jan-2017:  NAXIS1 created from AOI Width, NAXIS2 created from AOI Height\n\nWe're trying to explore how to rotate the image as displayed by FV so as a test I'm going to reverse these asssignments\n\n30-Jan-2017 Pavol reported this was NOT helpful so I've reversed them back the original mapping"
      # "34 rows x 80 characters =  2720 bytes\n23040 bytes (required block size) - 2720 =  20320 bytes which when divided by 80 characters per comment row requires\n\n254 more rows.  One of these is used up by the \"END\" row, leaving 253 rows of requiremed comments"
      # "Dec by 1\nfor \"END\" Row"
      # "2880 Bytes (FITS Header BLock size)x 8 = 23040 Bytes\n512 Byte (sector size) x 25 = 23040 Bytes\n\n2880 Bytes / 80 characters (bytes) per line = 36 lines\n\n23040 Bytes / 80 = 288 lines - 36 (first header already done) = 252 extra lines of 80 characters needed.\nThis will take the form of \"COMMENT + 73 spaces\" \n\n5660"
      n2 = call "SCMP FITS - Define FITS Keywords.vi"() -> ("Extension Comments"=w26:string[], "Extension  Keywords"=w27:string[], "Primary Comments"=w28:string[], "Primary Keywords"=w25:string[])  [unwired: 5 in, 3 out]
      n3 = Greater Than 0?(x="Image #") -> (x > 0?=w31:bool)
      n4 = global read "Globals.vi" "FITS BITPIX"() -> (w5:enum16{"16", "32"})
      n5 = case shown="True" w31 {
        tunnel: [w39 w41] -> w30
        tunnel: [w38 w40] -> w29
        tunnel: w25 -> [w39 _]
        tunnel: w28 -> [w38 _]
        tunnel: w27 -> [_ w41]
        tunnel: w26 -> [_ w40]
        frame False {
          # "Primary"
        }
        frame True {
          # "Extensions"
        }
      }
      n6 = for {
        tunnel: w30 -> [w44] mode=indexing
        tunnel: w29 -> [w48] mode=indexing
        tunnel: "FITS Header" -> [w49]
        tunnel: [w47] -> w13 mode=indexing
        tunnel: "Andor" -> [w46]
        tunnel: "Image #" -> [w45]
        tunnel: w5 -> [w43]
        tunnel: "FITS info" -> [w42]
        n7 = case shown="\"NAXIS3\"" w44 {
          selector: w44 -> [w54 w61 w68 w73 w78 w84 w90 w98 w105 w112 w118 w128 w134 w143 w147 w156 w167 w178 w184 w191 w199 w220 w227 w242 w254 w260 w268 w278 w289 w300 w310 w315 w323 w328 w335 w339 w347 w356 w388 w393 w398 w405 w409 w416 w424 w442 w449 w463 w468 w478 w488 w498 w508 w518 w526 w534 w541 w547 w552 w556 w565 w570 w574 w580 w591 w596 w603]
          tunnel: w49 -> [_ w58 _ _ _ _ _ _ _ _ _ w122 _ _ _ _ w164 w172 w180 w192 w200 _ w224 w244 w252 w258 w270 w276 _ w297 w307 _ _ _ _ _ w344 w353 w384 _ _ _ _ w413 _ _ _ _ _ w475 w485 w495 w505 w515 w522 w532 w538 _ _ w560 _ _ _ w577 w588 _ w599]
          tunnel: w48 -> [w52 w60 w67 w72 w77 w83 w89 w97 w104 w111 w117 w127 w133 w142 w146 w155 w166 w177 w183 w190 w198 w219 w226 w243 w253 w259 w269 w277 w288 w299 w309 w314 w322 w327 w334 w338 w346 w355 w387 w391 w397 w403 w408 w415 w423 w441 w450 w462 w467 w477 w487 w497 w507 w517 w525 w533 w540 w546 w550 w557 w564 w569 w573 w579 w590 w595 w602]
          tunnel: [w51 w59 w66 w71 w76 w82 w87 w96 w103 w110 w116 w126 w132 w141 w145 w154 w165 w176 w182 w189 w197 w218 w225 w240 w251 w257 w267 w279 w287 w298 w308 w313 w321 w326 w332 w337 w345 w354 w386 w390 w396 w404 w407 w414 w422 w440 w448 w461 w466 w476 w486 w496 w506 w516 w524 w530 w539 w545 w549 w555 w563 w568 w572 w578 w589 w594 w601] -> w47
          tunnel: [w50 w55 w65 w70 w75 w81 w88 w95 w102 w109 w115 w125 w131 w140 w144 w153 w163 w174 w181 w188 w196 w217 w222 w241 w250 w256 w266 w280 w286 w296 w304 w311 w320 w325 w333 w336 w342 w352 w385 w389 w395 w402 w406 w411 w421 w439 w447 w460 w464 w474 w484 w494 w504 w514 w523 w531 w536 w544 w548 w554 w561 w567 w571 w576 w584 w592 w600] -> _
          tunnel: w46 -> [_ _ _ _ _ _ _ w94 w101 w107 _ w121 _ w136 _ w150 w158 w169 _ _ _ _ _ _ _ _ _ _ _ _ _ _ _ _ _ _ _ _ _ _ _ _ _ _ _ w436 w451 _ _ _ _ _ _ _ _ _ _ _ _ _ _ _ _ _ _ _ _]
          tunnel: w45 -> [_ _ _ _ _ _ _ _ _ _ _ _ _ _ _ _ _ _ _ _ _ _ _ _ _ _ _ _ _ _ _ _ _ _ _ _ _ _ _ _ _ _ _ _ w419 _ _ _ _ _ _ _ _ _ _ _ _ _ _ _ _ _ _ _ _ _ _]
          tunnel: w43 -> [_ _ w64 _ _ w79 _ _ _ _ _ _ _ _ _ _ _ _ _ _ _ _ _ _ _ _ _ _ _ _ _ _ _ _ _ _ _ _ _ _ _ _ _ _ _ _ _ _ _ _ _ _ _ _ _ _ _ _ _ _ _ _ _ _ _ _ _]
          tunnel: w42 -> [_ _ _ _ _ _ _ _ _ _ _ _ _ _ _ _ _ _ _ _ _ w215 w221 _ _ _ _ _ _ _ _ _ w319 _ _ _ _ _ _ _ _ _ _ _ _ _ _ _ _ _ _ _ _ _ _ _ _ _ _ _ _ _ _ _ _ _ _]
          frame "", Default {
            n8 = call "FITS - Format FITS Keyword v2 .vi"("Keyword"=w54, "Value"="", "Comment"=w52) -> ("Formatted fits entry"=w51:string, "Length of line"=w50:i16)  [unwired: 1 in, 1 out]
          }
          frame "BEAM" {
            n9 = Unbundle By Name(w58) -> ("Beam Type (-1/1)"=w56:dbl)
            n10 = Number To Decimal String(number=w56) -> (decimal integer string=w57:string)  [unwired: 1 out]
            n11 = call "FITS - Format FITS Keyword v2 .vi"("Keyword"=w61, "Value"=w57, "Comment"=w60) -> ("Formatted fits entry"=w59:string, "Length of line"=w55:i16)  [unwired: 1 in, 1 out]
          }
          frame "BITPIX" {
            # "We decided in PDSS to sum multiple images at a given modulation state\nin order to sum more than 4 images we had to increase the bit depth\nfrom 16 bits to 32 bits"
            n12 = Format Into String(format string="%s", w64) -> (resulting string=w62:string)  [unwired: 2 in, 1 out]
            n13 = call "FITS - Format FITS Keyword v2 .vi"("Keyword"=w68, "Value"=w62, "Comment"=w67) -> ("Formatted fits entry"=w66:string, "Length of line"=w65:i16)  [unwired: 1 in, 1 out]
          }
          frame "BSCALE" {
            n14 = call "FITS - Format FITS Keyword v2 .vi"("Keyword"=w73, "Value"="1", "Comment"=w72) -> ("Formatted fits entry"=w71:string, "Length of line"=w70:i16)  [unwired: 1 in, 1 out]
          }
          frame "SOLARNET" {
            n15 = call "FITS - Format FITS Keyword v2 .vi"("Keyword"=w78, "Value"="-1", "Comment"=w77) -> ("Formatted fits entry"=w76:string, "Length of line"=w75:i16)  [unwired: 1 in, 1 out]
          }
          frame "BZERO" {
            n16 = case shown="\"32\"" w79 {
              tunnel: ["32768" ("Value") "2147483648" ("Value")] -> w80
              frame "16", Default {
              }
              frame "32" {
              }
            }
            n17 = call "FITS - Format FITS Keyword v2 .vi"("Keyword"=w84, "Value"=w80, "Comment"=w83) -> ("Formatted fits entry"=w82:string, "Length of line"=w81:i16)  [unwired: 1 in, 1 out]
          }
          frame "BUNIT" {
            n18 = call "FITS - Format FITS Keyword v2 .vi"("Keyword"=w90, "Value"="'ADU'", "Comment"=w89) -> ("Formatted fits entry"=w87:string, "Length of line"=w88:i16)  [unwired: 1 in, 1 out]
          }
          frame "CAM-BINX" {
            n19 = Unbundle By Name(w94) -> ("BDiv"=w93:u8)
            n20 = Number To Decimal String(number=w93) -> (decimal integer string=w92:string)  [unwired: 1 in]
            n21 = call "FITS - Format FITS Keyword v2 .vi"("Keyword"=w98, "Value"=w92, "Comment"=w97) -> ("Formatted fits entry"=w96:string, "Length of line"=w95:i16)  [unwired: 1 in, 1 out]
          }
          frame "CAM-BINY" {
            n22 = Unbundle By Name(w101) -> ("BDiv"=w99:u8)
            n23 = Number To Decimal String(number=w99) -> (decimal integer string=w100:string)  [unwired: 1 in]
            n24 = call "FITS - Format FITS Keyword v2 .vi"("Keyword"=w105, "Value"=w100, "Comment"=w104) -> ("Formatted fits entry"=w103:string, "Length of line"=w102:i16)  [unwired: 1 in, 1 out]
          }
          frame "CAM-ID" {
            # "camera position [1=straight,2=refletc]"
            n25 = Unbundle By Name(w107) -> ("Idx"=w106:i32)
            n26 = case shown="1" w106 {
              tunnel: ["1" ("string") "2" ("string")] -> w108
              frame 0, Default {
              }
              frame 1 {
              }
            }
            n27 = call "FITS - Format FITS Keyword v2 .vi"("Keyword"=w112, "Value"=w108, "Comment"=w111) -> ("Formatted fits entry"=w110:string, "Length of line"=w109:i16)  [unwired: 1 in, 1 out]
          }
          frame "CAM-PIXS" {
            n28 = call "FITS - Format FITS Keyword v2 .vi"("Keyword"=w118, "Value"="6.5", "Comment"=w117) -> ("Formatted fits entry"=w116:string, "Length of line"=w115:i16)  [unwired: 1 in, 1 out]
          }
          frame "CAM-POSI" {
            n29 = Unbundle By Name(w122) -> ("Camera PI (mm)"=w124:dbl[])
            n30 = Unbundle By Name(w121) -> ("Idx"=w123:i32)
            n31 = Index Array(array=w124, index=w123) -> (element=w120:dbl)
            n32 = Format Into String(format string="%7.3f", w120) -> (resulting string=w130:string)  [unwired: 2 in, 1 out]
            n33 = call "FITS - Format FITS Keyword v2 .vi"("Keyword"=w128, "Value"=w130, "Comment"=w127) -> ("Formatted fits entry"=w126:string, "Length of line"=w125:i16)  [unwired: 1 in, 1 out]
          }
          frame "CAM-ROX1" {
            n34 = call "FITS - Format FITS Keyword v2 .vi"("Keyword"=w134, "Value"="1", "Comment"=w133) -> ("Formatted fits entry"=w132:string, "Length of line"=w131:i16)  [unwired: 1 in, 1 out]
          }
          frame "CAM-ROX2" {
            n35 = Unbundle By Name(w136) -> ("AOI Width"=w138:i32)
            n36 = Number To Decimal String(number=w138, width (-)=i16 4) -> (decimal integer string=w137:string)
            n37 = call "FITS - Format FITS Keyword v2 .vi"("Keyword"=w143, "Value"=w137, "Comment"=w142) -> ("Formatted fits entry"=w141:string, "Length of line"=w140:i16)  [unwired: 1 in, 1 out]
          }
          frame "CAM-ROY1" {
            n38 = call "FITS - Format FITS Keyword v2 .vi"("Keyword"=w147, "Value"="1", "Comment"=w146) -> ("Formatted fits entry"=w145:string, "Length of line"=w144:i16)  [unwired: 1 in, 1 out]
          }
          frame "CAM-ROY2" {
            n39 = Unbundle By Name(w150) -> ("AOI Height"=w151:i32)
            n40 = Number To Decimal String(number=w151, width (-)=i16 4) -> (decimal integer string=w149:string)
            n41 = call "FITS - Format FITS Keyword v2 .vi"("Keyword"=w156, "Value"=w149, "Comment"=w155) -> ("Formatted fits entry"=w154:string, "Length of line"=w153:i16)  [unwired: 1 in, 1 out]
          }
          frame "CAM-SN" {
            w162 = "'" ("string")
            n42 = Unbundle By Name(w164) -> ("Camera Serial Number"=w160:string[])
            n43 = Unbundle By Name(w158) -> ("Idx"=w157:i32)
            n44 = Index Array(array=w160, index=w157) -> (element=w159:string)
            n45 = Concatenate Strings(w162, w159, w162) -> (w161:string)
            n46 = call "FITS - Format FITS Keyword v2 .vi"("Keyword"=w167, "Value"=w161, "Comment"=w166) -> ("Formatted fits entry"=w165:string, "Length of line"=w163:i16)  [unwired: 1 in, 1 out]
          }
          frame "CAM-TEMP" {
            n47 = Unbundle By Name(w169) -> ("Idx"=w168:i32)
            n48 = Unbundle By Name(w172) -> ("Camera Temp"=w171:dbl[])
            n49 = Index Array(array=w171, index=w168) -> (element=w170:dbl)
            n50 = Format Into String(format string="%6.2f", w170) -> (resulting string=w175:string)  [unwired: 2 in, 1 out]
            n51 = call "FITS - Format FITS Keyword v2 .vi"("Keyword"=w178, "Value"=w175, "Comment"=w177) -> ("Formatted fits entry"=w176:string, "Length of line"=w174:i16)  [unwired: 1 in, 1 out]
          }
          frame "COMMHEAD" {
            n52 = Unbundle By Name(w180) -> ("Comment"=w179:string)
            n53 = call "FITS - Format FITS Keyword v2 .vi"("Keyword"=w184, "Value"=w179, "Comment"=w183) -> ("Formatted fits entry"=w182:string, "Length of line"=w181:i16)  [unwired: 1 in, 1 out]
          }
          frame "COOKBOOK" {
            w187 = "'" ("string")
            n54 = Unbundle By Name(w192) -> ("Cookbook"=w186:string)
            n55 = Concatenate Strings(w187, w186, w187) -> (w185:string)
            n56 = call "FITS - Format FITS Keyword v2 .vi"("Keyword"=w191, "Value"=w185, "Comment"=w190) -> ("Formatted fits entry"=w189:string, "Length of line"=w188:i16)  [unwired: 1 in, 1 out]
          }
          frame "DATATYPE" {
            w195 = "'" ("string")
            n57 = disable-structure shown="Enabled" {
              disable-tunnel: w200 -> [w203 _]
              disable-tunnel: [w201 w214] -> w194
              frame Disabled {
                n58 = Unbundle By Name(w203) -> ("Data Type"=w202:T7)
                n59 = case shown="\"OBSE\"" w202 {
                  tunnel: ["DARK" "FLAT" "CALI" "OBSE" "ABSO" "AURE" "TARG" "OBJE" "HOLE" "LIVE"] -> w201
                  frame "LIVE", Default {
                  }
                  frame "DARK" {
                  }
                  frame "FLAT" {
                  }
                  frame "CALI" {
                  }
                  frame "OBSE" {
                  }
                  frame "ABSO" {
                  }
                  frame "AURE" {
                  }
                  frame "TARG" {
                  }
                  frame "OBJE" {
                  }
                  frame "HOLE" {
                  }
                }
              }
              frame Enabled {
                n60 = property on="Data Type" class="Enum (strict)"() -> ("RingText.Text"=w214:string)  [unwired: 2 in, 2 out]
              }
            }
            n61 = Concatenate Strings(w195, w194, w195) -> (w193:string)
            n62 = call "FITS - Format FITS Keyword v2 .vi"("Keyword"=w199, "Value"=w193, "Comment"=w198) -> ("Formatted fits entry"=w197:string, "Length of line"=w196:i16)  [unwired: 1 in, 1 out]
          }
          frame "DATE" {
            n63 = Unbundle By Name(w215) -> ("Date"=w216:string)
            n64 = call "FITS - Format FITS Keyword v2 .vi"("Keyword"=w220, "Value"=w216, "Comment"=w219) -> ("Formatted fits entry"=w218:string, "Length of line"=w217:i16)  [unwired: 1 in, 1 out]
          }
          frame "DATE-OBS" {
            # "FITS standard says that the DATE_OBS keyword is used for \nthe START of the observation"
            n65 = disable-structure shown="Enabled" {
              disable-tunnel: w224 -> [w229 w233]
              disable-tunnel: [w230 w236] -> w223
              disable-tunnel: w221 -> [_ _]
              frame Enabled {
                # "ten isty cas ako vo fits name"
                n66 = Unbundle By Name(w229) -> ("Time Start"=w228:timestamp)
                n67 = Format Date/Time String(time format string (%c)="%Y-%m-%dT%H:%M:%S", seconds (now)=w228) -> (date/time string=w230:string)  [unwired: 1 in]
              }
              frame Disabled {
                # "cas frame1 a zaokruhluje sa na sekundy"
                n68 = Unbundle By Name(w233) -> ("Time Stamp Array"=w234:timestamp[])
                n69 = Index Array(array=w234, index=0) -> (element=w232:timestamp)
                n70 = Format Date/Time String(time format string (%c)="%Y-%m-%dT%H:%M:%S", seconds (now)=w232) -> (date/time string=w236:string)  [unwired: 1 in]
              }
            }
            n71 = call "FITS - Format FITS Keyword v2 .vi"("Keyword"=w227, "Value"=w223, "Comment"=w226) -> ("Formatted fits entry"=w225:string, "Length of line"=w222:i16)  [unwired: 1 in, 1 out]
          }
          frame "DATE-END" {
            n72 = Unbundle By Name(w244) -> ("Time End"=w239:timestamp)
            n73 = Format Date/Time String(time format string (%c)="%Y-%m-%dT%H:%M:%S", seconds (now)=w239) -> (date/time string=w245:string)  [unwired: 1 in]
            n74 = call "FITS - Format FITS Keyword v2 .vi"("Keyword"=w242, "Value"=w245, "Comment"=w243) -> ("Formatted fits entry"=w240:string, "Length of line"=w241:i16)  [unwired: 1 in, 1 out]
          }
          frame "TIME-FR1" {
            n75 = Unbundle By Name(w252) -> ("Time Stamp Array"=w248:timestamp[])
            n76 = Index Array(array=w248, index=0) -> (element=w247:timestamp)
            n77 = Format Date/Time String(time format string (%c)="%H:%M:%S%3u", seconds (now)=w247) -> (date/time string=w255:string)  [unwired: 1 in]
            n78 = call "FITS - Format FITS Keyword v2 .vi"("Keyword"=w254, "Value"=w255, "Comment"=w253) -> ("Formatted fits entry"=w251:string, "Length of line"=w250:i16)  [unwired: 1 in, 1 out]
          }
          frame "TIME-FR2" {
            n79 = Unbundle By Name(w258) -> ("Time Stamp Array"=w263:timestamp[])
            n80 = Index Array(array=w263, index=1) -> (element=w262:timestamp)
            n81 = Format Date/Time String(time format string (%c)="%H:%M:%S%3u", seconds (now)=w262) -> (date/time string=w265:string)  [unwired: 1 in]
            n82 = call "FITS - Format FITS Keyword v2 .vi"("Keyword"=w260, "Value"=w265, "Comment"=w259) -> ("Formatted fits entry"=w257:string, "Length of line"=w256:i16)  [unwired: 1 in, 1 out]
          }
          frame "TIME-FR3" {
            n83 = Unbundle By Name(w270) -> ("Time Stamp Array"=w273:timestamp[])
            n84 = Index Array(array=w273, index=2) -> (element=w272:timestamp)
            n85 = Format Date/Time String(time format string (%c)="%H:%M:%S%3u", seconds (now)=w272) -> (date/time string=w275:string)  [unwired: 1 in]
            n86 = call "FITS - Format FITS Keyword v2 .vi"("Keyword"=w268, "Value"=w275, "Comment"=w269) -> ("Formatted fits entry"=w267:string, "Length of line"=w266:i16)  [unwired: 1 in, 1 out]
          }
          frame "TIME-FR4" {
            n87 = Unbundle By Name(w276) -> ("Time Stamp Array"=w283:timestamp[])
            n88 = Index Array(array=w283, index=3) -> (element=w282:timestamp)
            n89 = Format Date/Time String(time format string (%c)="%H:%M:%S%3u", seconds (now)=w282) -> (date/time string=w285:string)  [unwired: 1 in]
            n90 = call "FITS - Format FITS Keyword v2 .vi"("Keyword"=w278, "Value"=w285, "Comment"=w277) -> ("Formatted fits entry"=w279:string, "Length of line"=w280:i16)  [unwired: 1 in, 1 out]
          }
          frame "DETECTOR" {
            n91 = call "FITS - Format FITS Keyword v2 .vi"("Keyword"=w289, "Value"="'ANDOR NEO CAMERA'", "Comment"=w288) -> ("Formatted fits entry"=w287:string, "Length of line"=w286:i16)  [unwired: 1 in, 1 out]
          }
          frame "DIFFUSER" {
            n92 = Unbundle By Name(w297) -> ("Light Shapping Diffuser"=w294:T6)
            n93 = Build Array("'OUT OF BEAM'", "'IN BEAM'") -> (w295:string[])
            n94 = Index Array(array=w295, index=w294) -> (element=w293:string)
            n95 = call "FITS - Format FITS Keyword v2 .vi"("Keyword"=w300, "Value"=w293, "Comment"=w299) -> ("Formatted fits entry"=w298:string, "Length of line"=w296:i16)  [unwired: 1 in, 1 out]
          }
          frame "EXPTIME" {
            n96 = Unbundle By Name(w307) -> ("Exposure (s)"=w305:dbl)
            n97 = Multiply(x=1000.0, y=w305) -> (x*y=w302:dbl)
            n98 = Format Into String(format string="%_3f", w302) -> (resulting string=w306:string)  [unwired: 2 in, 1 out]
            n99 = call "FITS - Format FITS Keyword v2 .vi"("Keyword"=w310, "Value"=w306, "Comment"=w309) -> ("Formatted fits entry"=w308:string, "Length of line"=w304:i16)  [unwired: 1 in, 1 out]
          }
          frame "EXTEND" {
            n100 = call "FITS - Format FITS Keyword v2 .vi"("Keyword"=w315, "Value"="T", "Comment"=w314) -> ("Formatted fits entry"=w313:string, "Length of line"=w311:i16)  [unwired: 1 in, 1 out]
          }
          frame "FILENAME" {
            w318 = "'" ("string")
            n101 = Unbundle By Name(w319) -> ("File name"=w317:string)
            n102 = Concatenate Strings(w318, w317, w318) -> (w316:string)
            n103 = call "FITS - Format FITS Keyword v2 .vi"("Keyword"=w323, "Value"=w316, "Comment"=w322) -> ("Formatted fits entry"=w321:string, "Length of line"=w320:i16)  [unwired: 1 in, 1 out]
          }
          frame "FILTER" {
            n104 = disable-structure shown="SCMP==SCD" {
              disable-tunnel: ["'HAO Lyot 4-stage'" "'HAO Lyot 5-stage'"] -> w324
              frame condition #0 (active) {
              }
              frame condition #1 {
              }
            }
            n105 = call "FITS - Format FITS Keyword v2 .vi"("Keyword"=w328, "Value"=w324, "Comment"=w327) -> ("Formatted fits entry"=w326:string, "Length of line"=w325:i16)  [unwired: 1 in, 1 out]
          }
          frame "FLC-1" {
            n106 = call "FITS - Format FITS Keyword v2 .vi"("Keyword"=w335, "Value"="'+5.00,-5.00,+5.00,-5.00'", "Comment"=w334) -> ("Formatted fits entry"=w332:string, "Length of line"=w333:i16)  [unwired: 1 in, 1 out]
          }
          frame "FLC-2" {
            n107 = call "FITS - Format FITS Keyword v2 .vi"("Keyword"=w339, "Value"="'+5.00,-5.00,-5.00,+5.00'", "Comment"=w338) -> ("Formatted fits entry"=w337:string, "Length of line"=w336:i16)  [unwired: 1 in, 1 out]
          }
          frame "FOCUS" {
            n108 = Unbundle By Name(w344) -> ("Objective Lens Position (mm)"=w343:T12)
            n109 = Format Into String(format string="%5.2f", w343) -> (resulting string=w348:string)  [unwired: 2 in, 1 out]
            n110 = call "FITS - Format FITS Keyword v2 .vi"("Keyword"=w347, "Value"=w348, "Comment"=w346) -> ("Formatted fits entry"=w345:string, "Length of line"=w342:i16)  [unwired: 1 in, 1 out]
          }
          frame "FW-CALIB" {
            w351 = "'" ("string")
            n111 = disable-structure shown="SCMP==SCD" {
              disable-tunnel: w353 -> [w369 w382]
              disable-tunnel: [w367 w380] -> w350
              frame condition #0 {
                n112 = Unbundle By Name(w369) -> ("SCD Calibration Optics"=w368:T8)
                n113 = Build Array("LP0, I+Q", "LP90, I-Q", "LP45, I+U", "LP135, I-U" ("element"), "LCP, I+V" ("element"), "RCP, I-V" ("element"), "Dark" ("element"), "Clear" ("element"), "N/A" ("element")) -> (w357:string[])
                n114 = Index Array(array=w357, index=w368) -> (element=w367:string)
              }
              frame condition #1 (active) {
                n115 = Unbundle By Name(w382) -> ("COMP-S Calibration Wheel"=w381:T10)
                n116 = Build Array("Dark", "Clear", "Lens", "I+Q" ("element"), "I-Q" ("element"), "I+U" ("element"), "I-U" ("element"), "I+V" ("element"), "I-V" ("element")) -> (w372:string[])
                n117 = Index Array(array=w372, index=w381) -> (element=w380:string)
              }
            }
            n118 = Concatenate Strings(w351, w350, w351) -> (w349:string)
            n119 = call "FITS - Format FITS Keyword v2 .vi"("Keyword"=w356, "Value"=w349, "Comment"=w355) -> ("Formatted fits entry"=w354:string, "Length of line"=w352:i16)  [unwired: 1 in, 1 out]
          }
          frame "FW-WVLNG" {
            n120 = call "SCMP get wave from fw.vi"("FITS Header"=w384) -> ("element"=w383:string)  [unwired: 9 in, 1 out]
            n121 = call "FITS - Format FITS Keyword v2 .vi"("Keyword"=w388, "Value"=w383, "Comment"=w387) -> ("Formatted fits entry"=w386:string, "Length of line"=w385:i16)  [unwired: 1 in, 1 out]
          }
          frame "GCOUNT" {
            n122 = call "FITS - Format FITS Keyword v2 .vi"("Keyword"=w393, "Value"="1", "Comment"=w391) -> ("Formatted fits entry"=w390:string, "Length of line"=w389:i16)  [unwired: 1 in, 1 out]
          }
          frame "INSTRUME" {
            n123 = disable-structure shown="SCMP==SCD" {
              disable-tunnel: ["'COMP-S'" "'SCD'"] -> w394
              frame condition #0 (active) {
              }
              frame condition #1 {
              }
            }
            n124 = call "FITS - Format FITS Keyword v2 .vi"("Keyword"=w398, "Value"=w394, "Comment"=w397) -> ("Formatted fits entry"=w396:string, "Length of line"=w395:i16)  [unwired: 1 in, 1 out]
          }
          frame "LOCATION" {
            n125 = call "FITS - Format FITS Keyword v2 .vi"("Keyword"=w405, "Value"="'LOMNICKY PEAK OBSERVATORY'", "Comment"=w403) -> ("Formatted fits entry"=w404:string, "Length of line"=w402:i16)  [unwired: 1 in, 1 out]
          }
          frame "LEVEL" {
            n126 = call "FITS - Format FITS Keyword v2 .vi"("Keyword"=w409, "Value"="0", "Comment"=w408) -> ("Formatted fits entry"=w407:string, "Length of line"=w406:i16)  [unwired: 1 in, 1 out]
          }
          frame "MODC" {
            n127 = Unbundle By Name(w413) -> ("Mod Cycles"=w412:u16)
            n128 = Format Into String(format string="%d", w412) -> (resulting string=w417:string)  [unwired: 2 in, 1 out]
            n129 = call "FITS - Format FITS Keyword v2 .vi"("Keyword"=w416, "Value"=w417, "Comment"=w415) -> ("Formatted fits entry"=w414:string, "Length of line"=w411:i16)  [unwired: 1 in, 1 out]
          }
          frame "NAXIS" {
            n130 = Equal To 0?(x=w419) -> (x = 0?=w420:bool)
            n131 = case shown="False" w420 {
              tunnel: w424 -> [w427 w434]
              tunnel: w423 -> [w428 w433]
              tunnel: [w426 w432] -> w422
              tunnel: [w425 w431] -> w421
              frame False {
                # "All SCD Images have\n3 dimensions\nx-pixels\ny-pixels\npol state"
                n132 = call "FITS - Format FITS Keyword v2 .vi"("Keyword"=w427, "Value"="3", "Comment"=w428) -> ("Formatted fits entry"=w426:string, "Length of line"=w425:i16)  [unwired: 1 in, 1 out]
              }
              frame True {
                n133 = call "FITS - Format FITS Keyword v2 .vi"("Keyword"=w434, "Value"="0", "Comment"=w433) -> ("Formatted fits entry"=w432:string, "Length of line"=w431:i16)  [unwired: 1 in, 1 out]
              }
            }
          }
          frame "NAXIS1" {
            # "mh maj19 kamera na COMP-S je otocena o 90st\nmh jul19 -aj tak nakoniec netreba rotovat"
            n134 = disable-structure shown="SCMP==COMP, Default" {
              disable-tunnel: w436 -> [w444 w446]
              disable-tunnel: [w443 w445] -> w435
              frame condition #0 (active) {
                n135 = Unbundle By Name(w444) -> ("AOI Width"=w443:i32)
              }
              frame condition #1 {
                n136 = Unbundle By Name(w446) -> ("AOI Width"=w445:i32)
              }
            }
            n137 = Number To Decimal String(number=w435, width (-)=i16 4) -> (decimal integer string=w437:string)
            n138 = call "FITS - Format FITS Keyword v2 .vi"("Keyword"=w442, "Value"=w437, "Comment"=w441) -> ("Formatted fits entry"=w440:string, "Length of line"=w439:i16)  [unwired: 1 in, 1 out]
          }
          frame "NAXIS2" {
            # "mh maj19 kamera na COMP-S je otocena o 90st\nmh jul19 -aj tak nakoniec netreba rotovat"
            n139 = disable-structure shown="SCMP==COMP, Default" {
              disable-tunnel: w451 -> [w456 w458]
              disable-tunnel: [w455 w457] -> w452
              frame condition #0 (active) {
                n140 = Unbundle By Name(w456) -> ("AOI Height"=w455:i32)
              }
              frame condition #1 {
                n141 = Unbundle By Name(w458) -> ("AOI Height"=w457:i32)
              }
            }
            n142 = Number To Decimal String(number=w452, width (-)=i16 4) -> (decimal integer string=w453:string)
            n143 = call "FITS - Format FITS Keyword v2 .vi"("Keyword"=w449, "Value"=w453, "Comment"=w450) -> ("Formatted fits entry"=w448:string, "Length of line"=w447:i16)  [unwired: 1 in, 1 out]
          }
          frame "NAXIS3" {
            # "For a \"Snapshot\" NAXIS is 1\nFor cookbook based observations NAXIS is 4\n\nThe SCD modulator produces 4 modulation states\nhereafter know as A,B,C,D."
            n144 = call "FITS - Format FITS Keyword v2 .vi"("Keyword"=w463, "Value"="NAXIS", "Comment"=w462) -> ("Formatted fits entry"=w461:string, "Length of line"=w460:i16)  [unwired: 1 in, 1 out]
          }
          frame "NAXIS4" {
            # "SCD is a single camera instrument"
            n145 = call "FITS - Format FITS Keyword v2 .vi"("Keyword"=w468, "Value"="1", "Comment"=w467) -> ("Formatted fits entry"=w466:string, "Length of line"=w464:i16)  [unwired: 1 in, 1 out]
          }
          frame "NLC-1" {
            n146 = Unbundle By Name(w475) -> ("Tuning Voltages"=w471:dbl[])
            n147 = Index Array(array=w471, index=0) -> (element=w470:dbl)
            n148 = Format Into String(format string="%0.3f", w470) -> (resulting string=w469:string)  [unwired: 2 in, 1 out]
            n149 = call "FITS - Format FITS Keyword v2 .vi"("Keyword"=w478, "Value"=w469, "Comment"=w477) -> ("Formatted fits entry"=w476:string, "Length of line"=w474:i16)  [unwired: 1 in, 1 out]
          }
          frame "NLC-2" {
            n150 = Unbundle By Name(w485) -> ("Tuning Voltages"=w481:dbl[])
            n151 = Index Array(array=w481, index=1) -> (element=w480:dbl)
            n152 = Format Into String(format string="%0.3f", w480) -> (resulting string=w479:string)  [unwired: 2 in, 1 out]
            n153 = call "FITS - Format FITS Keyword v2 .vi"("Keyword"=w488, "Value"=w479, "Comment"=w487) -> ("Formatted fits entry"=w486:string, "Length of line"=w484:i16)  [unwired: 1 in, 1 out]
          }
          frame "NLC-3" {
            n154 = Unbundle By Name(w495) -> ("Tuning Voltages"=w491:dbl[])
            n155 = Index Array(array=w491, index=2) -> (element=w490:dbl)
            n156 = Format Into String(format string="%0.3f", w490) -> (resulting string=w489:string)  [unwired: 2 in, 1 out]
            n157 = call "FITS - Format FITS Keyword v2 .vi"("Keyword"=w498, "Value"=w489, "Comment"=w497) -> ("Formatted fits entry"=w496:string, "Length of line"=w494:i16)  [unwired: 1 in, 1 out]
          }
          frame "NLC-4" {
            n158 = Unbundle By Name(w505) -> ("Tuning Voltages"=w501:dbl[])
            n159 = Index Array(array=w501, index=3) -> (element=w500:dbl)
            n160 = Format Into String(format string="%0.3f", w500) -> (resulting string=w499:string)  [unwired: 2 in, 1 out]
            n161 = call "FITS - Format FITS Keyword v2 .vi"("Keyword"=w508, "Value"=w499, "Comment"=w507) -> ("Formatted fits entry"=w506:string, "Length of line"=w504:i16)  [unwired: 1 in, 1 out]
          }
          frame "NLC-5" {
            n162 = Unbundle By Name(w515) -> ("Tuning Voltages"=w511:dbl[])
            n163 = Index Array(array=w511, index=4) -> (element=w510:dbl)
            n164 = Format Into String(format string="%0.3f", w510) -> (resulting string=w509:string)  [unwired: 2 in, 1 out]
            n165 = call "FITS - Format FITS Keyword v2 .vi"("Keyword"=w518, "Value"=w509, "Comment"=w517) -> ("Formatted fits entry"=w516:string, "Length of line"=w514:i16)  [unwired: 1 in, 1 out]
          }
          frame "OBSERVER" {
            w521 = "'" ("string")
            n166 = Unbundle By Name(w522) -> ("Observer"=w520:string)
            n167 = Concatenate Strings(w521, w520, w521) -> (w519:string)
            n168 = call "FITS - Format FITS Keyword v2 .vi"("Keyword"=w526, "Value"=w519, "Comment"=w525) -> ("Formatted fits entry"=w524:string, "Length of line"=w523:i16)  [unwired: 1 in, 1 out]
          }
          frame "OBS_PROG" {
            w529 = "'" ("string")
            n169 = Unbundle By Name(w532) -> ("Comment"=w528:string)
            n170 = Concatenate Strings(w529, w528, w529) -> (w527:string)
            n171 = call "FITS - Format FITS Keyword v2 .vi"("Keyword"=w534, "Value"=w527, "Comment"=w533) -> ("Formatted fits entry"=w530:string, "Length of line"=w531:i16)  [unwired: 1 in, 1 out]
          }
          frame "OCC-SIZE" {
            n172 = Unbundle By Name(w538) -> ("Occulter size"=w537:dbl)
            n173 = Format Into String(format string="%5.2f", w537) -> (resulting string=w542:string)  [unwired: 2 in, 1 out]
            n174 = call "FITS - Format FITS Keyword v2 .vi"("Keyword"=w541, "Value"=w542, "Comment"=w540) -> ("Formatted fits entry"=w539:string, "Length of line"=w536:i16)  [unwired: 1 in, 1 out]
          }
          frame "ORIGIN" {
            n175 = call "FITS - Format FITS Keyword v2 .vi"("Keyword"=w547, "Value"="'AISAS'", "Comment"=w546) -> ("Formatted fits entry"=w545:string, "Length of line"=w544:i16)  [unwired: 1 in, 1 out]
          }
          frame "PCOUNT" {
            n176 = call "FITS - Format FITS Keyword v2 .vi"("Keyword"=w552, "Value"="0", "Comment"=w550) -> ("Formatted fits entry"=w549:string, "Length of line"=w548:i16)  [unwired: 1 in, 1 out]
          }
          frame "ROTPOS" {
            n177 = Unbundle By Name(w560) -> ("FOV Rotation (deg)"=w559:dbl)
            n178 = Format Into String(format string="%5.1f", w559) -> (resulting string=w558:string)  [unwired: 2 in, 1 out]
            n179 = call "FITS - Format FITS Keyword v2 .vi"("Keyword"=w556, "Value"=w558, "Comment"=w557) -> ("Formatted fits entry"=w555:string, "Length of line"=w554:i16)  [unwired: 1 in, 1 out]
          }
          frame "SIMPLE" {
            # "FITS Standard Keyword (scott is not sure what it means)"
            n180 = call "FITS - Format FITS Keyword v2 .vi"("Keyword"=w565, "Value"="T", "Comment"=w564) -> ("Formatted fits entry"=w563:string, "Length of line"=w561:i16)  [unwired: 1 in, 1 out]
          }
          frame "TELESCOP" {
            n181 = call "FITS - Format FITS Keyword v2 .vi"("Keyword"=w570, "Value"="'ZEISS 200/3000 CORONAGRAPH'", "Comment"=w569) -> ("Formatted fits entry"=w568:string, "Length of line"=w567:i16)  [unwired: 1 in, 1 out]
          }
          frame "TIMESYS" {
            n182 = call "FITS - Format FITS Keyword v2 .vi"("Keyword"=w574, "Value"="'UTC'", "Comment"=w573) -> ("Formatted fits entry"=w572:string, "Length of line"=w571:i16)  [unwired: 1 in, 1 out]
          }
          frame "TUNEDLAY" {
            n183 = Unbundle By Name(w577) -> ("Tuning Delay (ms)"=w583:dbl)
            n184 = Format Into String(format string="%d", w583) -> (resulting string=w581:string)  [unwired: 2 in, 1 out]
            n185 = call "FITS - Format FITS Keyword v2 .vi"("Keyword"=w580, "Value"=w581, "Comment"=w579) -> ("Formatted fits entry"=w578:string, "Length of line"=w576:i16)  [unwired: 1 in, 1 out]
          }
          frame "WAVELENG" {
            n186 = Unbundle By Name(w588) -> ("Wavelength (nm)"=w587:dbl)
            n187 = Format Into String(format string="%0.3f", w587) -> (resulting string=w585:string)  [unwired: 2 in, 1 out]
            n188 = call "FITS - Format FITS Keyword v2 .vi"("Keyword"=w591, "Value"=w585, "Comment"=w590) -> ("Formatted fits entry"=w589:string, "Length of line"=w584:i16)  [unwired: 1 in, 1 out]
          }
          frame "XTENSION" {
            n189 = call "FITS - Format FITS Keyword v2 .vi"("Keyword"=w596, "Value"="'IMAGE'", "Comment"=w595) -> ("Formatted fits entry"=w594:string, "Length of line"=w592:i16)  [unwired: 1 in, 1 out]
          }
          frame "XPOSURE" {
            n190 = Unbundle By Name(w599) -> ("Acc Exposure (s)"=w598:dbl)
            n191 = Format Into String(format string="%_3f", w598) -> (resulting string=w604:string)  [unwired: 2 in, 1 out]
            n192 = call "FITS - Format FITS Keyword v2 .vi"("Keyword"=w603, "Value"=w604, "Comment"=w602) -> ("Formatted fits entry"=w601:string, "Length of line"=w600:i16)  [unwired: 1 in, 1 out]
          }
        }
      }
      n193 = Array Size(array=w13) -> (size(s)=w9:i32)
      "Header Rows" <- w9
      n194 = Divide(x=23040, y=80) -> (x/y=w10:dbl)
      n195 = Subtract(x=w10, y=w9) -> (x-y=w8:dbl)
      n196 = Decrement(x=w8) -> (x-1=w7:dbl)
      "Required COMMENT Rows" <- w7
      n197 = Format Into String(format string="COMMENT%73s", "") -> (resulting string=w16:string)  [unwired: 2 in, 1 out]
      n198 = for {
        N: w7 -> [_]
        tunnel: w16 -> [w34]
        tunnel: [w34] -> w15 mode=indexing
      }
      n199 = Format Into String(format string="END%77s", "") -> (resulting string=w20:string)  [unwired: 2 in, 1 out]
      n200 = Build Array (concatenate)(w13, w15, w20) -> (w22:string[])
      "FITS Header" <- w22
      n201 = for {
        tunnel: w22 -> [w36] mode=indexing
        shift-right: [w37] -> w19
        shift-left: "" -> [w35]
        n202 = Concatenate Strings(w35, w36) -> (w37:string)
      }
      "23040 Byte Header" <- w19
      n203 = String Length(string=w19) -> (length=→"final header byte length":i32)
    }
    frame Error {
    }
  }
  "error out" <- w1
